vi "Amp_PS_gets.vi"(0 "error in (no error)":errorcluster, 1 "delay before read (ms)":u32=500, 2 "Amp PS address":refnum<visa-resource-name>) -> (3 "output cluster":T1, 4 "status":bool, 5 "current, A":dbl, 6 "voltage, V":dbl)   [LabVIEW 2010]
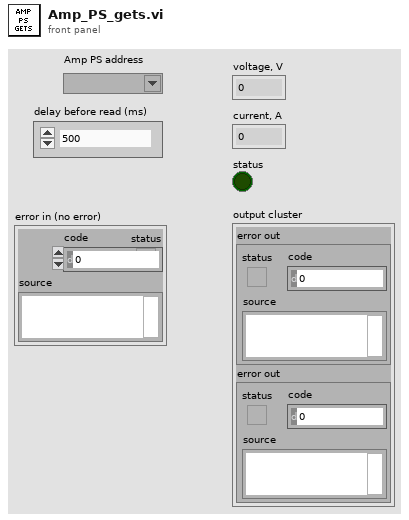
[diagram p1: front panel]
types:
  T1 = cluster{"error out":errorcluster, "error out":errorcluster}
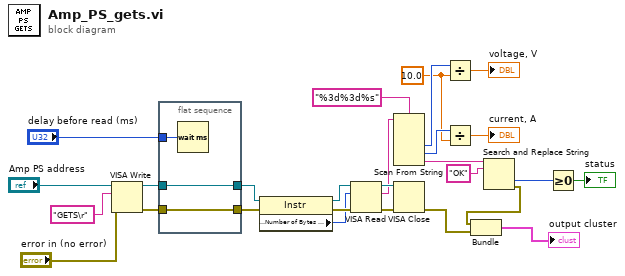
[diagram p0: block diagram]
diagram:
  w9 = 10.0 ("y")
  n1 = VISA Write(VISA resource name="Amp PS address", write buffer="GETS\r", error in (no error)="error in (no error)") -> (VISA resource name out=w23:refnum<visa-resource-name>, error out=w25:errorcluster)  [unwired: 1 out]
  n2 = flat-sequence {
    tunnel: w25 -> [w29]
    tunnel: [w29] -> w24
    tunnel: w23 -> [w28]
    tunnel: [w28] -> w22
    tunnel: "delay before read (ms)" -> [w30]
    frame #0 {
      n3 = Wait (ms)(milliseconds to wait=w30) -> ()  [unwired: 1 out]
    }
  }
  n4 = property class="Instr"(reference=w22, error in=w24) -> (reference out=w21:refnum<visa-resource-name>, error out=w20:errorcluster, "Serial Settings:Number of Bytes at Serial Port"=w19:u32)
  n5 = VISA Read(VISA resource name=w21, byte count=w19, error in (no error)=w20) -> (VISA resource name out=w26:refnum<visa-resource-name>, read buffer=w12:string, error out=w27:errorcluster)  [unwired: 1 out]
  n6 = Scan From String(format string="%3d%3d%s", input string=w12) -> (output 1=w11:i32, output 2=w10:i32, output 3=w6:string)  [unwired: 5 in, 3 out]
  n7 = VISA Close(VISA resource name=w26, error in (no error)=w27) -> (error out=w2:errorcluster)
  n8 = Divide(x=w11, y=w9) -> (x/y=→"voltage, V":dbl)
  n9 = Divide(x=w10, y=w9) -> (x/y=→"current, A":dbl)
  n10 = Search and Replace String(input string=w6, search string="OK" ("true string")) -> (offset past replacement=w14:i32, error out=w3:errorcluster)  [unwired: 6 in, 2 out]
  n11 = Bundle("error out"=w3, "error out"=w2) -> (→"output cluster":T1)  [unwired: 1 in]
  n12 = Greater Or Equal To 0?(x=w14) -> (x >= 0?=→"status":bool)
